vi "Vision Research Phantom Series PhInt PhImProc.vi"(0 "Camera Number (1)":u32=1, 2 "pPixel In":u16[](array[numeric]), 5 "Error In (no error)":errorcluster, 7 "pBMIH":T5, 9 "pOpt":T1 {"FilterCode" items=["PREWITT_3X3_V"=1, "PREWITT_3X3_H"=2, "SOBEL_3X3_V"=3, "SOBEL_3X3_H"=4, "LAPLACIAN_3X3"=5, "LAPLACIAN_5X5"=6, "GAUSSIAN_3X3"=7, "GAUSSIAN_5X5"=8, "HIPASS_3x3"=9, "HIPASS_5x5"=10, "SHARPEN_3X3"=11, "USERFILTER"=-1]; "Rotate" min=-90 max=90 step=1; "Saturation" min=-100 max=100 step=1; "Contrast" min=-100 max=100 step=1; "Bright" min=-100 max=100 step=1}) -> (14 "Camera Number out":u32=1, 16 "pPixel":u16[](array[numeric]), 19 "Error Out":errorcluster)   [LabVIEW 2013, in "VRI.lvlib"]
doc: "PhInt.DLL\n\nPhImProc\nPhImProc(PBITMAPINFOHEADER pBMIH, PBYTE pPixel, PIMPROCOPTIONS pOpt);\n\nParameters Description\npBMIH Source and destination header of the processed image.\npPixel Source and destination pixel array of the processed image.\npOpt Structure describing the operations to do\nReturn Void\nComments This function provide the image processing for 8 and 16 bits, gray or color. \n The order of applying the processings is:\n 1. WBView (White Balance correction)\n 2. Contrast, Bright, Gamma\n 3. Saturation\n 4. Flip\n 5. Rotate\n 6. Filter\n To change the order of processings, call the function multiple times with \n one processing selected each time.\n\n\nWritten by:\nBLOOMY CONTROLS, INC\nWINDSOR, CT 06095, USA\n860-298-9925\nwww.bloomy.com\nV1.0.0\nMay, 2004"
uses:
  VRI.lvlib
  _Type Defs/BITMAPINFOHEADER.ctl
  _Type Defs/PhInt IMPROCOPTIONS.ctl
  _Type Defs/PhInt WBGAIN.ctl
  _Type Defs/FilterCode.ctl
  _Type Defs/IMFILTER.ctl
  Phantom DLLs/PhInt.dll
panel:
  # "For instructions on the use of this VI, press Ctrl+H to display the help window and move the mouse over the icon, controls, and indicators"
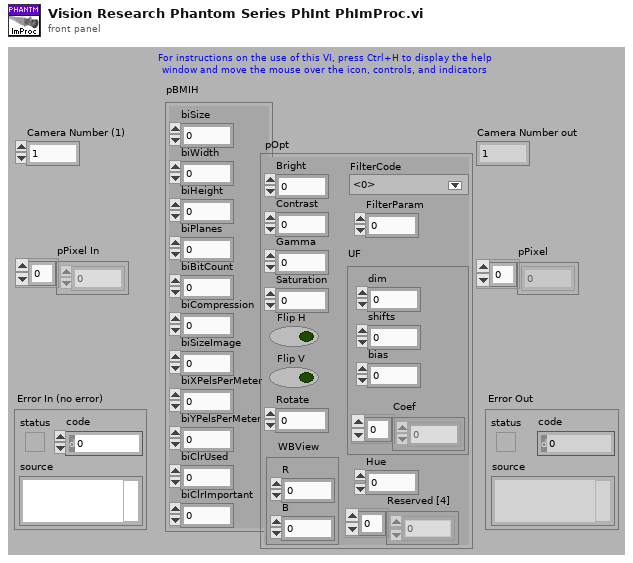
[diagram p1: front panel]
types:
  T1 = typedef "VRI.lvlib/PhInt IMPROCOPTIONS.ctl" = cluster{"Bright":i32, "Contrast":i32, "Gamma":sgl, "Saturation":i32, "Flip H":bool, "Flip V":bool, "Rotate":i32, "WBView":T2, "FilterCode":T3, "FilterParam":i32, "UF":T4, "Hue":i32, "Reserved [4]":i32[]}
  T2 = typedef "VRI.lvlib/PhInt WBGAIN.ctl" = cluster{"R":sgl, "B":sgl}
  T3 = typedef "VRI.lvlib/FilterCode.ctl" = i32
  T4 = typedef "VRI.lvlib/IMFILTER.ctl" = cluster{"dim":i32, "shifts":i32, "bias":i32, "Coef":i32[]}
  T5 = typedef "VRI.lvlib/BITMAPINFOHEADER.ctl" = cluster{"biSize":u32, "biWidth":i32, "biHeight":i32, "biPlanes":u16, "biBitCount":u16, "biCompression":u32, "biSizeImage":u32, "biXPelsPerMeter":i32, "biYPelsPerMeter":i32, "biClrUsed":u32, "biClrImportant":u32}
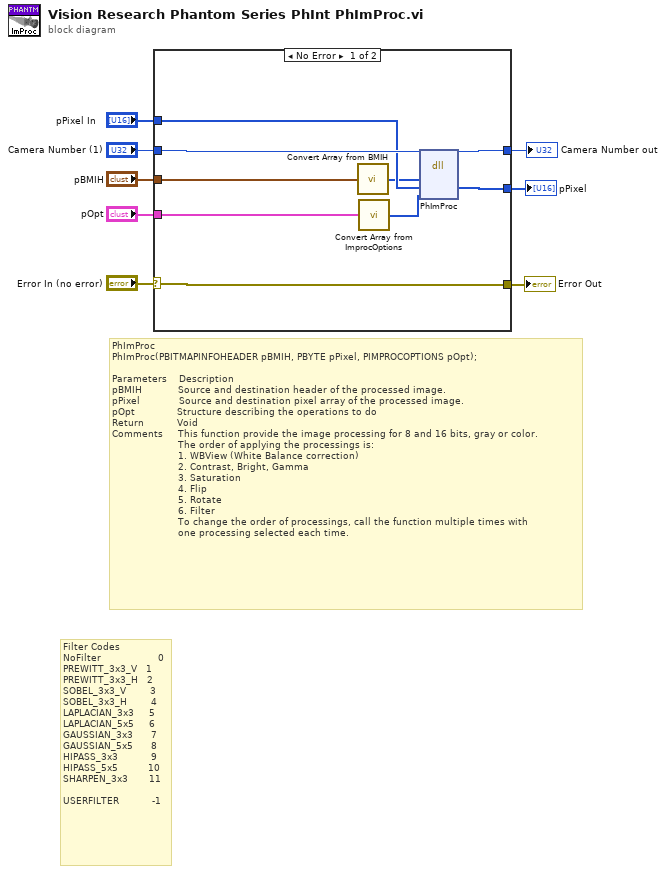
[diagram p0: block diagram]
diagram:
  # "Filter Codes\nNoFilter                   0\nPREWITT_3x3_V   1\nPREWITT_3x3_H   2\nSOBEL_3x3_V        3\nSOBEL_3x3_H        4\nLAPLACIAN_3x3     5\nLAPLACIAN_5x5     6\nGAUSSIAN_3x3      7\nGAUSSIAN_5x5      8\nHIPASS_3x3           9\nHIPASS_5x5          10\nSHARPEN_3x3       11\n\nUSERFILTER           -1"
  # "PhImProc\nPhImProc(PBITMAPINFOHEADER pBMIH, PBYTE pPixel, PIMPROCOPTIONS pOpt);\n\nParameters    Description\npBMIH            Source and destination header of the processed image.\npPixel             Source and destination pixel array of the processed image.\npOpt              Structure describing the operations to do\nReturn           Void\nComments     This function provide the image processing for 8 and 16 bits, gray or color. \n                      The order of applying the processings is:\n                      1. WBView (White Balance correction)\n                      2. Contrast, Bright, Gamma\n                      3. Saturation\n                      4. Flip\n                      5. Rotate\n                      6. Filter\n                      To change the order of processings, call the function multiple times with \n                      one processing selected each time."
  n1 = case shown="No Error" "Error In (no error)" {
    selector: "Error In (no error)" -> [w16 w19]
    tunnel: [w16 w19] -> w7
    tunnel: "Camera Number (1)" -> [w15 w18]
    tunnel: [w15 w18] -> w5
    tunnel: [w14 w17] -> w4
    tunnel: "pBMIH" -> [w13 _]
    tunnel: "pOpt" -> [w12 _]
    tunnel: "pPixel In" -> [w11 w17]
    frame No Error {
      n2 = call "Convert Array from BMIH.vi"("BITMAPINFOHEADER"=w13) -> ("Array"=w10:u8[])
      n3 = call "Convert Array from ImprocOptions.vi"("IMPROCOPTIONS"=w12) -> ("Array"=w9:i32[])
      n4 = dll-call lib="C:/Projects/SDK/32-bit/Vision Research Phantom Series Labview Driver/Phantom DLLs/PhInt.dll" fn="PhImProc"("pBMIH"=w10, "pPixel"=w11, "pOpt"=w9) -> ("pPixel"=w14:u16[])  [unwired: 5 in, 3 out]
    }
    frame Error {
    }
  }
  "Error Out" <- w7
  "Camera Number out" <- w5
  "pPixel" <- w4
